vi "samples to waveform.vi"(8 "Channel ID (row)":i32, 9 "ad_scan_desc":T1={"sample_rate"=0.001, "clock_rate"=0.0, "prehist"=0, "posthist"=500, "ticks_per_run"=0, "bytes_per_run"=0, "samples_per_run"=0, "flags"=0, "sd_res[0]"=0, "sd_res[1]"=0, "sd_res[2]"=0, "sd_res[3]"=0, "sd_res[4]"=0, "sd_res[5]"=0, "sd_res[6]"=0, "sd_res[7]"=0, "sd_res[8]"=0, "sd_res[9]"=0, "sd_res[10]"=0, "sd_res[11]"=0}, 10 "chav in":T2[](array[typedef]), 11 "buffer in":sgl[](array[numeric])) -> (3 "Waveform":waveform(sgl))   [LabVIEW 2021, in "libad4.lvlib"]
uses:
  <userlib>/libad4/libad4.lvlib
  <userlib>/libad4/controls/ad scan cha desc.ctl
  <userlib>/libad4/controls/ad scan desc.ctl
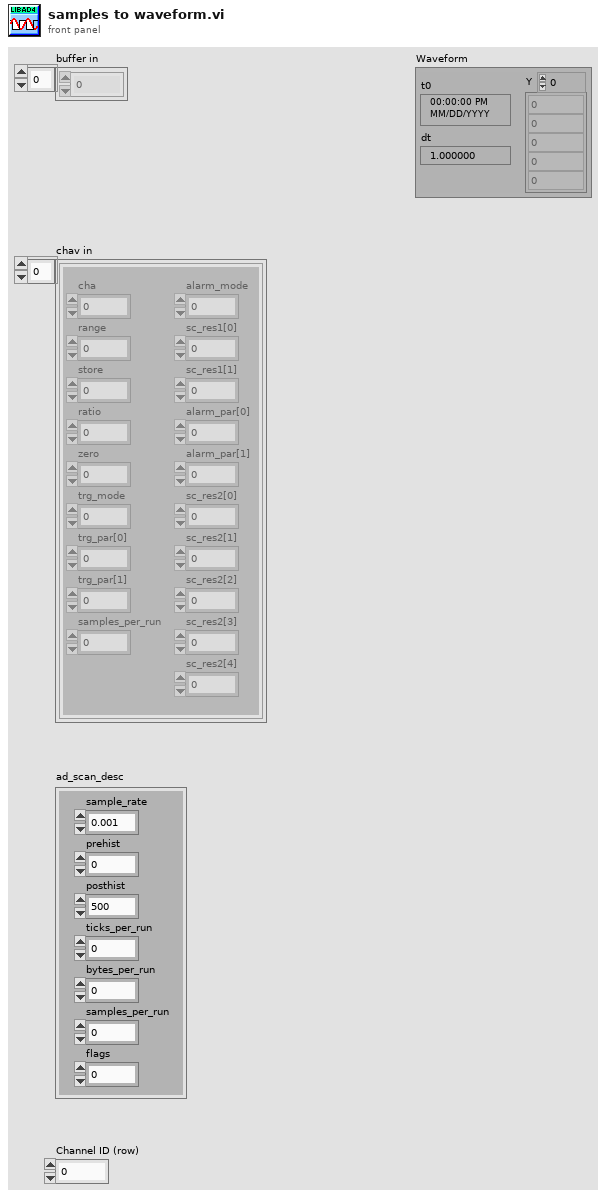
[diagram p1: front panel]
types:
  T1 = typedef "libad4.lvlib/ad scan desc.ctl" = cluster{"sample_rate":dbl, "clock_rate":dbl, "prehist":u64, "posthist":u64, "ticks_per_run":u32, "bytes_per_run":u32, "samples_per_run":u32, "flags":u32, "sd_res[0]":u32, "sd_res[1]":u32, "sd_res[2]":u32, "sd_res[3]":u32, "sd_res[4]":u32, "sd_res[5]":u32, "sd_res[6]":u32, "sd_res[7]":u32, "sd_res[8]":u32, "sd_res[9]":u32, "sd_res[10]":u32, "sd_res[11]":u32}
  T2 = typedef "libad4.lvlib/ad scan cha desc.ctl" = cluster{"cha":i32, "range":i32, "store":i32, "ratio":i32, "zero":u32, "trg_mode":u8, "alarm_mode":u8, "sc_res1[0]":u8, "sc_res1[1]":u8, "trg_par[0]":u32, "trg_par[1]":u32, "samples_per_run":i32, "alarm_par[0]":u32, "alarm_par[1]":u32, "sc_res2[0]":u32, "sc_res2[1]":u32, "sc_res2[2]":u32, "sc_res2[3]":u32, "sc_res2[4]":u32}
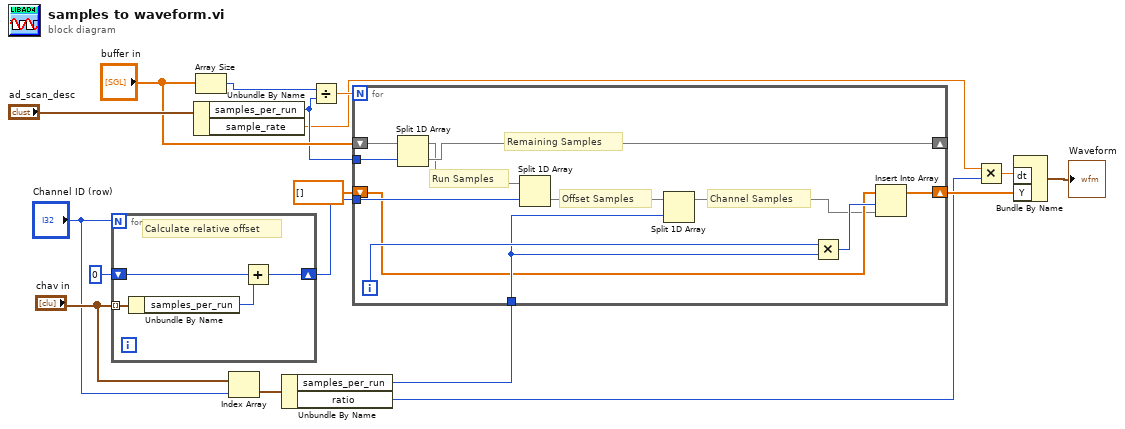
[diagram p0: block diagram]
diagram:
  n1 = for {
    N: "Channel ID (row)" -> [_]
    tunnel: "chav in" -> [w21] mode=indexing
    shift-right: [w18] -> w10
    shift-left: 0 -> [w19]
    # "Calculate relative offset"
    n2 = Unbundle By Name(w21) -> ("samples_per_run"=w20:i32)
    n3 = Add(x=w19, y=w20) -> (x+y=w18:i32)
  }
  n4 = Unbundle By Name("ad_scan_desc") -> ("samples_per_run"=w11:u32, "sample_rate"=w2:dbl)
  n5 = Array Size(array="buffer in") -> (size(s)=w16:i32)
  n6 = Index Array(array="chav in", index="Channel ID (row)") -> (element=w7:T2)
  n7 = Unbundle By Name(w7) -> ("samples_per_run"=w6:i32, "ratio"=w1:i32)
  n8 = Divide(x=w16, y=w11) -> (x/y=w15:dbl)
  n9 = for {
    N: w15 -> [_]
    tunnel: w11 -> [w32]
    shift-right: [w31] -> _
    shift-left: "buffer in" -> [w33]
    tunnel: w10 -> [w29]
    tunnel: w6 -> [w26]
    shift-right: [w24] -> w4
    shift-left: sgl[] [] -> [w23]
    i -> [w27]
    # "Channel Samples"
    # "Offset Samples"
    # "Remaining Samples"
    # "Run Samples"
    n10 = Split 1D Array(array=w33, index=w32) -> (first subarray=w30:sgl[], second subarray=w31:sgl[])
    n11 = Split 1D Array(array=w30, index=w29) -> (second subarray=w28:sgl[])  [unwired: 1 out]
    n12 = Split 1D Array(array=w28, index=w26) -> (first subarray=w22:sgl[])  [unwired: 1 out]
    n13 = Multiply(x=w27, y=w26) -> (x*y=w25:i32)
    n14 = Insert Into Array(array=w23, index=w25, new element=w22) -> (w24:sgl[])
  }
  n15 = Multiply(x=w2, y=w1) -> (x*y=w3:dbl)
  n16 = Bundle By Name("dt"=w3, "Y"=w4) -> (→"Waveform":waveform(sgl))  [unwired: 1 in]
